vi "9225 3Ch Analog Input.vi"(1 "9225 I/O":T1={"9225 AI0"="NI 9225/AI0", "9225 AI1"="NI 9225/AI1", "9225 AI2"="NI 9225/AI2"}) -> (0 "Packets":u64[](array[numeric]))   [LabVIEW 2010]
uses:
  <vilib>/eio/EIONode/EIONode.xnode
  <vilib>/rvi/eio/nirviEIOImplementation/nirviEIOImplementation.xnode
  <vilib>/rvi/eio/common/nirviEmuClasses.ctl
  <vilib>/rvi/eio/common/nirviEmuTemplateMethod_noerrors.vi
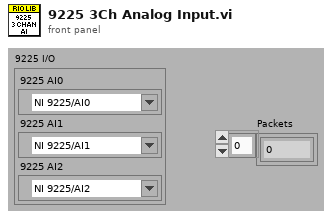
[diagram p1: front panel]
types:
  T1 = cluster{"9225 AI0":refnum<k21>, "9225 AI1":refnum<k21>, "9225 AI2":refnum<k21>}
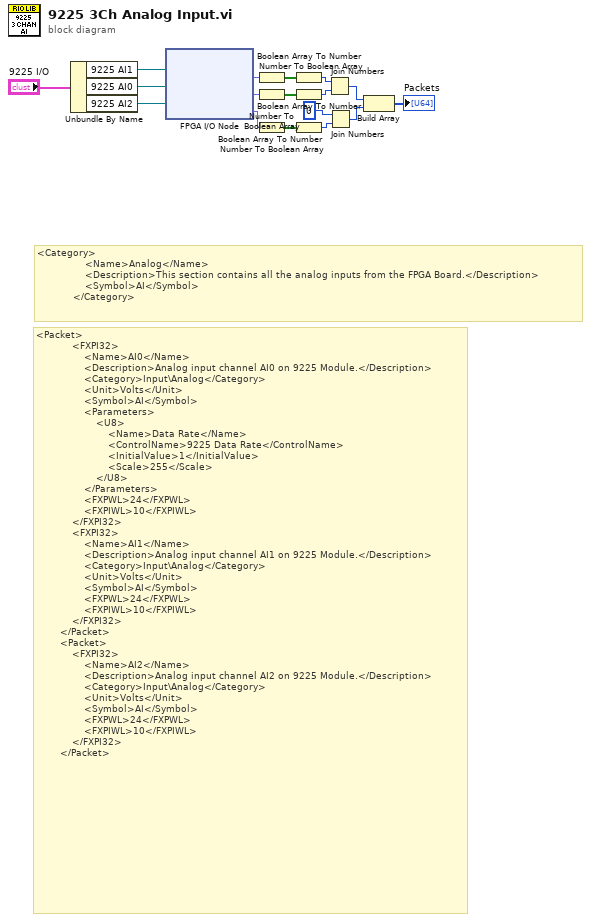
[diagram p0: block diagram]
diagram:
  # "<Category>\n                <Name>Analog</Name>\n                <Description>This section contains all the analog inputs from the FPGA Board.</Description>\n                <Symbol>AI</Symbol>\n            </Category>"
  # "<Packet>\n            <FXPI32>\n                <Name>AI0</Name>\n                <Description>Analog input channel AI0 on 9225 Module.</Description>\n                <Category>Input\\Analog</Category>\n                <Unit>Volts</Unit>\n                <Symbol>AI</Symbol>\n                <Parameters>\n                    <U8>\n                        <Name>Data Rate</Name>\n                        <ControlName>9225 Data Rate</ControlName>\n                        <InitialValue>1</InitialValue>\n                        <Scale>255</Scale>\n                    </U8>\n                </Parameters>\n                <FXPWL>24</FXPWL>\n                <FXPIWL>10</FXPIWL>\n            </FXPI32>\n            <FXPI32>\n                <Name>AI1</Name>\n                <Description>Analog input channel AI1 on 9225 Module.</Description>\n                <Category>Input\\Analog</Category>\n                <Unit>Volts</Unit>\n                <Symbol>AI</Symbol>\n                <FXPWL>24</FXPWL>\n                <FXPIWL>10</FXPIWL>\n            </FXPI32>\n        </Packet>\n        <Packet>\n            <FXPI32>\n                <Name>AI2</Name>\n                <Description>Analog input channel AI2 on 9225 Module.</Description>\n                <Category>Input\\Analog</Category>\n                <Unit>Volts</Unit>\n                <Symbol>AI</Symbol>\n                <FXPWL>24</FXPWL>\n                <FXPIWL>10</FXPIWL>\n            </FXPI32>\n        </Packet>"
  n1 = Unbundle By Name("9225 I/O") -> ("9225 AI1"=w6:refnum<k21>, "9225 AI0"=w7:refnum<k21>, "9225 AI2"=w8:refnum<k21>)
  n2 = xnode "FPGA I/O Node"("FPGA I/O In"=w6, "FPGA I/O In"=w7, "FPGA I/O In"=w8) -> ("I/O Item"=w12:fxp<+/-,24,10>, "I/O Item"=w14:fxp<+/-,24,10>, "I/O Item"=w13:fxp<+/-,24,10>)  [unwired: 3 out]
  n3 = Number To Boolean Array(number=w12) -> (Boolean array=w9:bool[])
  n4 = Number To Boolean Array(number=w14) -> (Boolean array=w10:bool[])
  n5 = Number To Boolean Array(number=w13) -> (Boolean array=w11:bool[])
  n6 = Boolean Array To Number(Boolean array=w9) -> (number=w15:u32)
  n7 = Boolean Array To Number(Boolean array=w10) -> (number=w16:u32)
  n8 = Boolean Array To Number(Boolean array=w11) -> (number=w17:u32)
  n9 = Join Numbers(hi=w15, lo=w16) -> ((hi.lo)=w4:u64)
  n10 = Join Numbers(hi=u32 0, lo=w17) -> ((hi.lo)=w5:u64)
  n11 = Build Array(w4, w5) -> (→"Packets":u64[])
